vi "8P_top_level.vi"() -> (0 "DAQ Error":errorcluster)   [LabVIEW 2020]
doc: "Use this plug-in with the Nathan 7609 data acquisition system"
uses:
  <vilib>/Instr/_visa.llb/VISA Find Search Mode.ctl
  Globals/Meas_global.vi
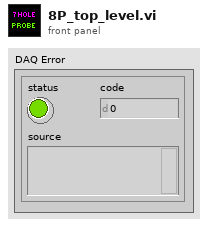
[diagram p1: front panel]
types:
  T1 = typedef "Analysis_info_cluster.ctl" = cluster{"Colour":u32, "Inst type":T2, "Inst name":string, "Symbol":string, "Code name":string, "Extra Info":string, "Inst Array":T3, "Extra Titles":string[], "Extra Values":string[], "U":dbl, "u^2":dbl, "u^3":dbl, "u^4":dbl, "Skew_u":dbl, "Kurt_u":dbl, "Sd Error in Mean":dbl, "% u'/U":dbl, "X":dbl, "Y":dbl, "Z":dbl, "Timescale integral Estimate":dbl, "Sd Error in Variance":dbl, "Calib File":path, "Calib Constants":dbl[], "Output Position":bool, "Stats":enum16{"None", "Basic", "Full"}, "Av Sampling Rate":dbl, "Av No of Samples":dbl, "Total Meas Time (s)":dbl, "ADAM Ch Name":string, "Max value":dbl, "Min value":dbl, "Req Sample Rate Hz":dbl, "Sync Delay Time (s)":dbl, "Ch No":i16, "Device":string, "Use Latest Calib":bool, "Port":string, "Metadata Ch Names":string[], "Metadata Ch Values":string[], "Label":string}
  T2 = typedef "Inst_type.ctl" = enum16{"Propeller anemometer", "Raw voltage", "Pressure Transducer", "Pitot-static tube", "Preston tube", "Hot wire", "Cross wire 1", "Cross wire 2", "Generic Linear", "Generic Polynomial", "Generic BackPoly", "Fast FID", "Thermocouple", "Cold wire", "Pulsed Wire", "LDA Vel", "LDA Tran time", "LDA Arr time", "Microphone"}
  T3 = typedef "Instrument_Array.ctl" = enum16{"PWA", "LDA", "Analogue"}
  T4 = typedef "Device ID port info.ctl" = cluster{"Ch No":i16[], "Req Sampling Rate":dbl[], "Port":string, "Index":i32[]}
  T5 = typedef "Setup.ctl" = enum16{"Run Program", "Show Setup", "Save Current Setup", "Setup Front Panel"}
  T6 = typedef "VISA Find Search Mode.ctl" = u32
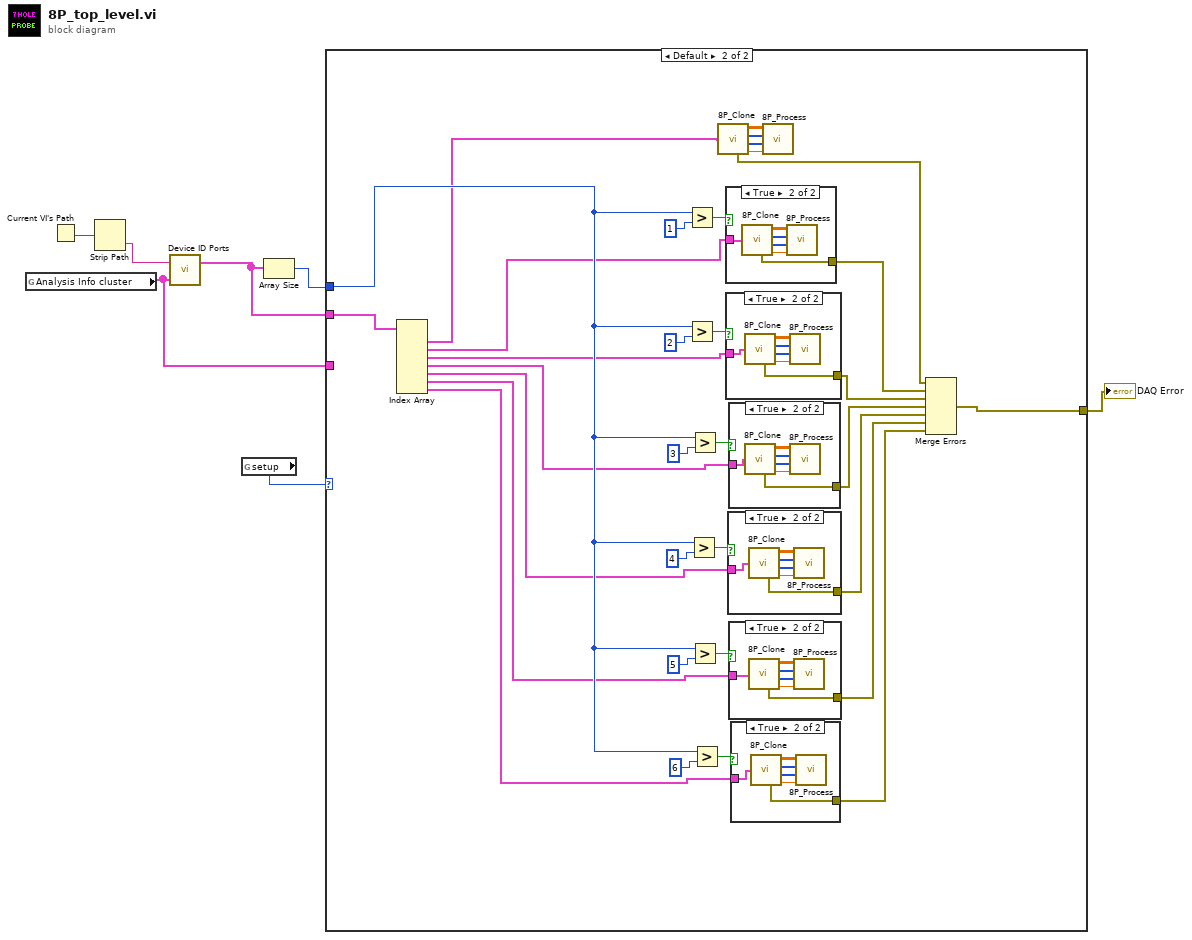
[diagram p0: block diagram]
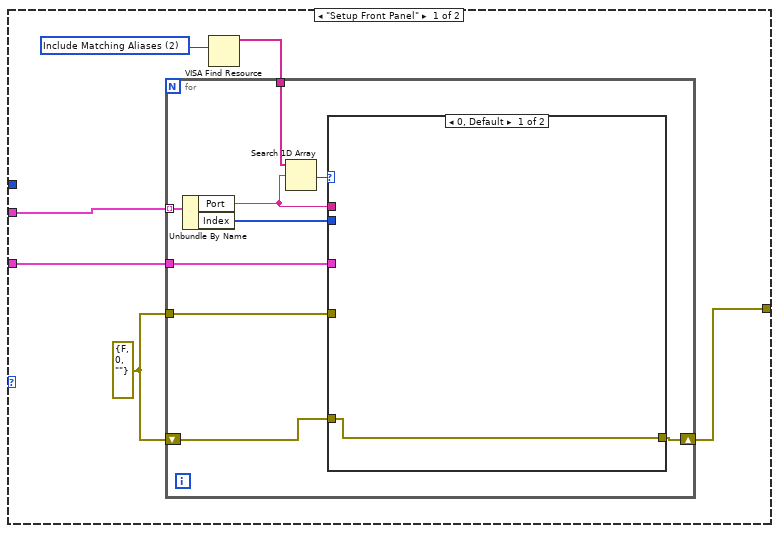
[diagram p2: hidden frame]
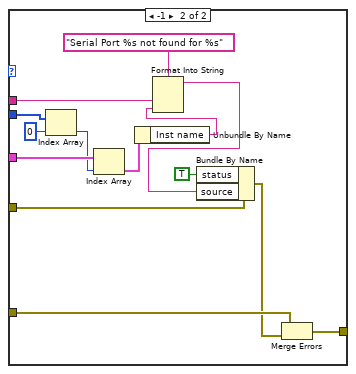
[diagram p3: hidden frame]
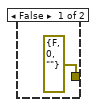
[diagram p4: hidden frame]
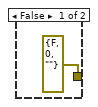
[diagram p5: hidden frame]
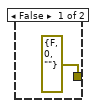
[diagram p6: hidden frame]
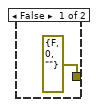
[diagram p7: hidden frame]
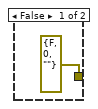
[diagram p8: hidden frame]
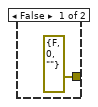
[diagram p9: hidden frame]
diagram:
  n1 = global read "Meas_global.vi" "Analysis Info cluster"() -> (w1:T1[])
  n2 = Current VI's Path() -> (path=w4:path)
  n3 = Strip Path(path=w4) -> (name=w3:string)  [unwired: 1 out]
  n4 = call "Device ID Ports.vi"("Analysis Info cluster"=w1, "Device ID"=w3) -> ("Device port info"=w2:T4[])  [unwired: 1 out]
  n5 = global read "Meas_global.vi" "setup"() -> (w5:T5)
  n6 = Array Size(array=w2) -> (size(s)=w7:i32)
  n7 = case shown="Default" w5 {
    tunnel: w2 -> [w13 w70]
    tunnel: w7 -> [_ w57]
    tunnel: [w12 w44] -> w6
    tunnel: w1 -> [w8 _]
    frame "Setup Front Panel" {
      w11 = T6 2 items=["Canonical Names Only"=0, "Aliases Only"=1, "Include Matching Aliases"=2, "Include All Aliases"=4] ("Search Mode")
      w9 = errorcluster {"status"=FALSE, "code"=0, "source"=""} ("error IO")
      n8 = VISA Find Resource(10:w11) -> (3:w10:string[])  [unwired: 1 in, 3 out]
      n9 = for {
        tunnel: w13 -> [w22] mode=indexing
        shift-right: [w20] -> w12
        shift-left: w9 -> [w21]
        tunnel: w10 -> [w19]
        tunnel: w9 -> [w17]
        tunnel: w8 -> [w14]
        n10 = Unbundle By Name(w22) -> ("Port"=w16:string, "Index"=w15:i32[])
        n11 = Search 1D Array(1D array=w19, element=w16) -> (index of element=w18:i32)  [unwired: 1 in]
        n12 = case shown="0, Default" w18 {
          tunnel: w21 -> [w23 w36]
          tunnel: [w23 w37] -> w20
          tunnel: w17 -> [_ w33]
          tunnel: w16 -> [_ w32]
          tunnel: w15 -> [_ w30]
          tunnel: w14 -> [_ w28]
          frame 0, Default {
          }
          frame -1 {
            n13 = Index Array(array=w30, index=0) -> (element=w27:i32)
            n14 = Index Array(array=w28, index=w27) -> (element=w26:T1)
            n15 = Unbundle By Name(w26) -> ("Inst name"=w25:string)
            n16 = Format Into String(format string="Serial Port %s not found for %s", w32, w25) -> (resulting string=w24:string)  [unwired: 2 in, 1 out]
            n17 = Bundle By Name(cluster=w33, "status"=TRUE, "source"=w24) -> (w34:errorcluster)
            n18 = Merge Errors(w36, w34) -> (w37:errorcluster)
          }
        }
      }
    }
    frame Default {
      n19 = Index Array(array=w70) -> (element #1=w39:T4, element #2=w56:T4, element #3=w55:T4, element #4=w54:T4, element #5=w53:T4, element #6=w52:T4, element #7=w51:T4)  [unwired: 7 in]
      n20 = Greater?(x=w57, y=1) -> (0:w68:bool)
      n21 = Greater?(x=w57, y=2) -> (0:w67:bool)
      n22 = Greater?(x=w57, y=4) -> (0:w63:bool)
      n23 = Greater?(x=w57, y=3) -> (0:w64:bool)
      n24 = Greater?(x=w57, y=5) -> (0:w60:bool)
      n25 = Greater?(x=w57, y=6) -> (0:w59:bool)
      n26 = call "8P_Clone.vi"("Single 8HP"=w39) -> ("DAQ Error"=w38:errorcluster, "All samples out"=w40:sgl[][], "Ch No"=w41:i16[], "Index"=w42:i32[], "Sampling Rate Hz"=w43:dbl)  [unwired: 1 in]
      n27 = case shown="True" w68 {
        tunnel: w56 -> [_ w107]
        tunnel: [errorcluster {"status"=FALSE, "code"=0, "source"=""} ("DAQ Error") w108] -> w50
        frame False {
        }
        frame True {
          n28 = call "8P_Clone.vi"("Single 8HP"=w107) -> ("DAQ Error"=w108:errorcluster, "All samples out"=w112:sgl[][], "Ch No"=w111:i16[], "Index"=w110:i32[], "Sampling Rate Hz"=w109:dbl)  [unwired: 1 in]
          n29 = call "8P_Process.vi"("All samples in"=w112, "8HP Ch No"=w111, "Analysis info Index"=w110, "Sampling Rate"=w109) -> ()  [unwired: 4 in]
        }
      }
      n30 = case shown="True" w67 {
        tunnel: w55 -> [_ w100]
        tunnel: [errorcluster {"status"=FALSE, "code"=0, "source"=""} ("DAQ Error") w101] -> w49
        frame False {
        }
        frame True {
          n31 = call "8P_Clone.vi"("Single 8HP"=w100) -> ("DAQ Error"=w101:errorcluster, "All samples out"=w103:sgl[][], "Ch No"=w104:i16[], "Index"=w105:i32[], "Sampling Rate Hz"=w102:dbl)  [unwired: 1 in]
          n32 = call "8P_Process.vi"("All samples in"=w103, "8HP Ch No"=w104, "Analysis info Index"=w105, "Sampling Rate"=w102) -> ()  [unwired: 4 in]
        }
      }
      n33 = case shown="True" w63 {
        tunnel: w53 -> [_ w86]
        tunnel: [errorcluster {"status"=FALSE, "code"=0, "source"=""} ("DAQ Error") w87] -> w47
        frame False {
        }
        frame True {
          n34 = call "8P_Clone.vi"("Single 8HP"=w86) -> ("DAQ Error"=w87:errorcluster, "All samples out"=w88:sgl[][], "Ch No"=w89:i16[], "Index"=w90:i32[], "Sampling Rate Hz"=w91:dbl)  [unwired: 1 in]
          n35 = call "8P_Process.vi"("All samples in"=w88, "8HP Ch No"=w89, "Analysis info Index"=w90, "Sampling Rate"=w91) -> ()  [unwired: 4 in]
        }
      }
      n36 = case shown="True" w64 {
        tunnel: w54 -> [_ w93]
        tunnel: [errorcluster {"status"=FALSE, "code"=0, "source"=""} ("DAQ Error") w94] -> w48
        frame False {
        }
        frame True {
          n37 = call "8P_Clone.vi"("Single 8HP"=w93) -> ("DAQ Error"=w94:errorcluster, "All samples out"=w98:sgl[][], "Ch No"=w97:i16[], "Index"=w96:i32[], "Sampling Rate Hz"=w95:dbl)  [unwired: 1 in]
          n38 = call "8P_Process.vi"("All samples in"=w98, "8HP Ch No"=w97, "Analysis info Index"=w96, "Sampling Rate"=w95) -> ()  [unwired: 4 in]
        }
      }
      n39 = case shown="True" w60 {
        tunnel: w52 -> [_ w79]
        tunnel: [errorcluster {"status"=FALSE, "code"=0, "source"=""} ("DAQ Error") w80] -> w46
        frame False {
        }
        frame True {
          n40 = call "8P_Clone.vi"("Single 8HP"=w79) -> ("DAQ Error"=w80:errorcluster, "All samples out"=w84:sgl[][], "Ch No"=w83:i16[], "Index"=w82:i32[], "Sampling Rate Hz"=w81:dbl)  [unwired: 1 in]
          n41 = call "8P_Process.vi"("All samples in"=w84, "8HP Ch No"=w83, "Analysis info Index"=w82, "Sampling Rate"=w81) -> ()  [unwired: 4 in]
        }
      }
      n42 = case shown="True" w59 {
        tunnel: w51 -> [_ w73]
        tunnel: [errorcluster {"status"=FALSE, "code"=0, "source"=""} ("DAQ Error") w72] -> w45
        frame False {
        }
        frame True {
          n43 = call "8P_Clone.vi"("Single 8HP"=w73) -> ("DAQ Error"=w72:errorcluster, "All samples out"=w74:sgl[][], "Ch No"=w75:i16[], "Index"=w76:i32[], "Sampling Rate Hz"=w77:dbl)  [unwired: 1 in]
          n44 = call "8P_Process.vi"("All samples in"=w74, "8HP Ch No"=w75, "Analysis info Index"=w76, "Sampling Rate"=w77) -> ()  [unwired: 4 in]
        }
      }
      n45 = call "8P_Process.vi"("All samples in"=w40, "8HP Ch No"=w41, "Analysis info Index"=w42, "Sampling Rate"=w43) -> ()  [unwired: 4 in]
      n46 = Merge Errors(w38, w50, w49, w48, w47, w46, w45) -> (w44:errorcluster)
    }
  }
  "DAQ Error" <- w6
